vi "Set Scan Settings.vi"(10 "Scan Settings":T1, 11 "Start Open Loop Scan Command in":refnum<class "Start Open Loop Scan Command.lvclass">) -> (3 "Start Open Loop Scan Command out":refnum<class "Start Open Loop Scan Command.lvclass">)   [LabVIEW 2015, in "Start Open Loop Scan Command.lvclass"]
uses:
  Start Open Loop Scan Command.lvclass
  Typedefs/Scan Settings.ctl
  Typedefs/FAMT Typedefs.lvlib
  Typedefs/Waveform Types.ctl
  Typedefs/Waveform Settings.ctl
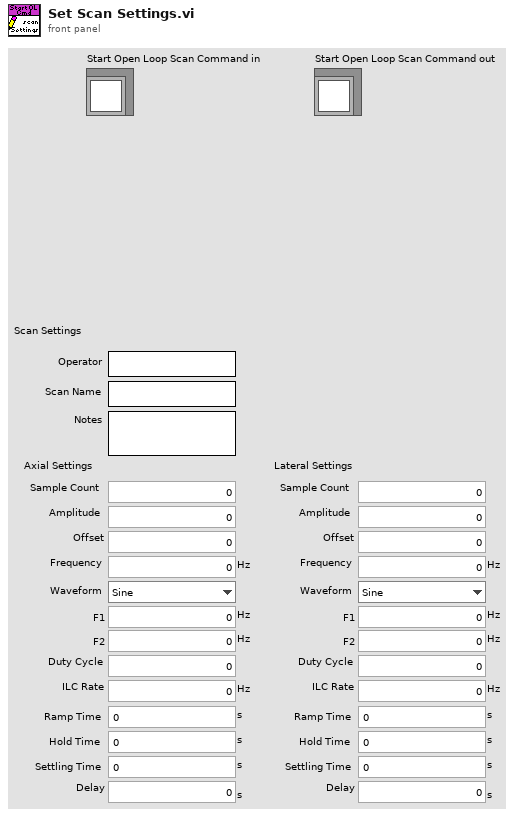
[diagram p1: front panel]
types:
  T1 = typedef "FAMT Typedefs.lvlib/Scan Settings.ctl" = cluster{"Operator":string, "Scan Name":string, "Notes":string, "Axial Settings":T2, "Lateral Settings":T2}
  T2 = typedef "FAMT Typedefs.lvlib/Waveform Settings.ctl" = cluster{"Sample Count":u32, "Amplitude":dbl, "Offset":dbl, "Frequency":dbl[unit], "Waveform":T3, "F1":dbl[unit], "F2":dbl[unit], "Duty Cycle":dbl, "ILC Rate":dbl[unit], "Ramp Time":dbl[unit], "Hold Time":dbl[unit], "Settling Time":dbl[unit], "Delay":dbl[unit]}
  T3 = typedef "FAMT Typedefs.lvlib/Waveform Types.ctl" = enum16{"Sine", "Triangle", "Square", "Sawtooth", "Chirp", "Gaussian", "Trapezoid"}
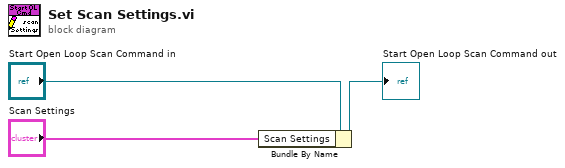
[diagram p0: block diagram]
diagram:
  n1 = Bundle By Name(cluster="Start Open Loop Scan Command in", "Scan Settings"="Scan Settings") -> (→"Start Open Loop Scan Command out":refnum<class "Start Open Loop Scan Command.lvclass">)
